vi "Actor Core.vi"(8 "error in":errorcluster, 11 "Test Actor in":refnum<class "Example Actor.lvclass">) -> (0 "error out":errorcluster, 3 "Actor out":refnum<class "Actor.lvclass">)   [LabVIEW 2020, in "Example Actor.lvlib" / "Example Actor.lvclass"]
doc: "(<B>Filename</B>: Actor Framework.lvlib:Actor.lvclass:Actor Core.vi)\n\nReceives messages to the actor, reacts to them, and initiates any error handling that may shut the actor down.\n\nDescendant classes may override this VI to append parallel tasks for the actor to complete while it handles messages. Overrides use the Call Parent Method node."
uses:
  Example Actor.lvclass
  C:/Program Files/National Instruments/LabVIEW 2020/vi.lib/ActorFramework/Actor/Actor.lvclass
  <vilib>/ActorFramework/Actor/Actor.lvclass
  Example Actor.lvclass/Example Actor.ctl
  <vilib>/ActorFramework/Actor/Actor.lvclass/Actor.ctl
  <vilib>/ActorFramework/Message Enqueuer/Message Enqueuer.lvclass/Message Enqueuer.ctl
  <vilib>/ActorFramework/Message Enqueuer/Init from Existing Queue.vi
  <vilib>/ActorFramework/Message Enqueuer/Enqueue.vi
  <vilib>/ActorFramework/Stop Msg/Stop Msg.lvclass
  C:/Program Files/National Instruments/LabVIEW 2020/vi.lib/ActorFramework/Message/Message.lvclass
  <vilib>/ActorFramework/Message Priority Queue/Priority Enqueue.vi
  <vilib>/ActorFramework/Message Enqueuer/Message Enqueuer.lvclass
  <vilib>/MGI/Monitored Actor/Monitored Actor/Monitored Actor/Monitored Actor.lvclass
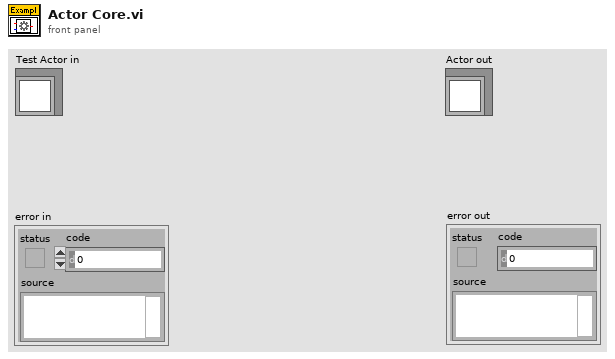
[diagram p1: front panel]
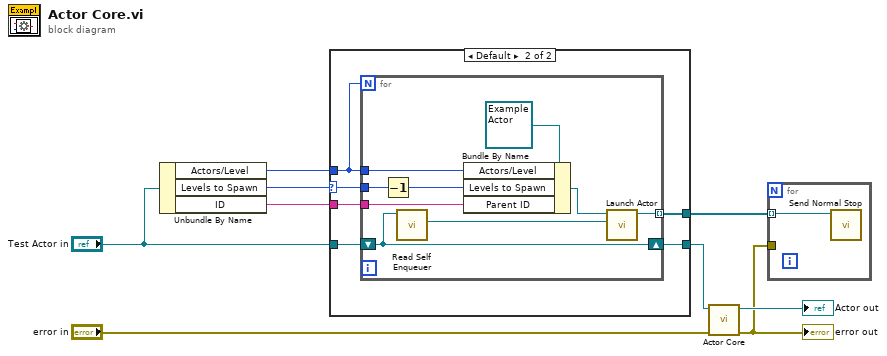
[diagram p0: block diagram]
diagram:
  n1 = Unbundle By Name("Test Actor in") -> ("Actors/Level"=w7:i32, "Levels to Spawn"=w1:i32, "ID"=w2:string)
  n2 = case shown="Default" w1 {
    selector: w1 -> [_ w12]
    tunnel: w7 -> [_ w11]
    tunnel: "Test Actor in" -> [w10 w16]
    tunnel: [w10 w15] -> w5
    tunnel: [_ w14] -> w4
    tunnel: w2 -> [_ w13]
    frame 0 {
    }
    frame Default {
      n3 = for {
        N: w11 -> [_]
        shift-right: [w25] -> w15
        shift-left: w16 -> [w25]
        tunnel: [w23] -> w14 mode=indexing
        tunnel: w13 -> [w20]
        tunnel: w12 -> [w19]
        tunnel: w11 -> [w17]
        n4 = Decrement(x=w19) -> (x-1=w18:i32)
        n5 = call <vilib>:"Read Self Enqueuer.vi"("Actor"=w25) -> ("Self Enqueuer"=w24:refnum<class "Message Enqueuer.lvclass">)  [unwired: 10 in]
        n6 = Bundle By Name(cluster=refnum<class "Example Actor.lvclass"> refnum ("Test Actor.lvclass"), "Actors/Level"=w17, "Levels to Spawn"=w18, "Parent ID"=w20) -> (w21:refnum<class "Example Actor.lvclass">)
        n7 = call <vilib>:"Launch Actor.vi"("Actor-to-Caller Enqueuer"=w24, "Actor"=w21) -> ("Caller-To-Actor Enqueuer"=w23:refnum<class "Message Enqueuer.lvclass">)  [unwired: 8 in, 1 out]
      }
    }
  }
  n8 = call-parent "Actor Core.vi"("error in"="error in", "Actor in"=w5) -> ("error out"=w3:errorcluster, "Actor out"=→"Actor out":refnum<class "Actor.lvclass">)  [unwired: 8 in]
  "error out" <- w3
  n9 = for {
    tunnel: w4 -> [w26] mode=indexing
    tunnel: w3 -> [_]
    n10 = call <vilib>:"Send Normal Stop.vi"("Message Enqueuer"=w26) -> ()  [unwired: 10 in, 1 out]
  }
